vi "Get Arguments.vi"(7 "Function Name":string, 8 "Error In":errorcluster, 11 "OPI Ref":refnum<data-value>) -> (0 "Error Out":errorcluster, 1 "Args Array":string[][](array[string]), 3 "OPI Ref":refnum<data-value>)   [LabVIEW 2012, in "OPI.lvclass"]
doc: "Get the arguments defined for a function. \n\nThe arguments are provided in the format of valid pythonic declaration and 2D array of strings representing argument and pythonic value pairs.\n\n You can keep these representation to reuse them or call them on the PES. This way you can quickly switch between predefined value sets."
uses:
  OPI.lvclass
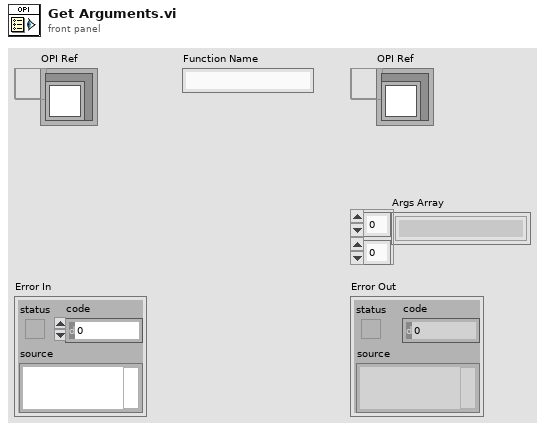
[diagram p1: front panel]
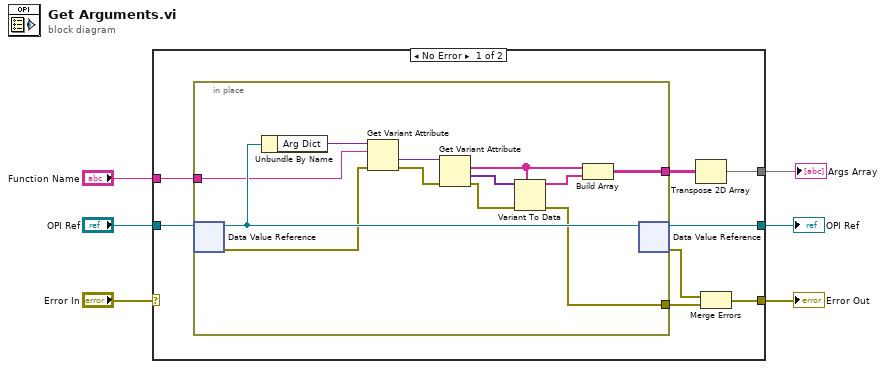
[diagram p0: block diagram]
diagram:
  n1 = case shown="No Error" "Error In" {
    selector: "Error In" -> [_ w27]
    tunnel: "OPI Ref" -> [w14 _]
    tunnel: "Function Name" -> [w13 _]
    tunnel: [w7 _] -> w3
    tunnel: [w9 w27] -> w2
    tunnel: [w8 _] -> w1
    frame No Error {
      n2 = in-place {
        in-place-border: w13 -> [w22]
        in-place-border: [w19] -> w12
        in-place-border: [w17] -> w11
        n3 = in-place-dvr #1(w14) -> (w26:refnum<class "OPI.lvclass">, w18:errorcluster)
        n4 = Unbundle By Name(w26) -> ("Arg Dict"=w23:variant)
        n5 = Get Variant Attribute(Variant=w23, name=w22, error in=w18) -> (value=w24:variant, error out=w25:errorcluster)  [unwired: 1 in, 2 out]
        n6 = Get Variant Attribute(Variant=w24, error in=w25) -> (names=w16:string[], values=w21:variant[], error out=w20:errorcluster)  [unwired: 2 in, 1 out]
        n7 = Variant To Data(error in=w20, type=w16, Variant=w21) -> (data=w15:string[], error out=w17:errorcluster)
        n8 = Build Array(w16, w15) -> (w19:string[][])
        n9 = in-place-dvr #1(w26) -> (w8:refnum<data-value>, w10:errorcluster)
      }
      n10 = Transpose 2D Array(2D array=w12) -> (transposed array=w7:string[][])
      n11 = Merge Errors(w10, w11) -> (w9:errorcluster)
    }
    frame Error {
    }
  }
  "Error Out" <- w2
  "OPI Ref" <- w1
  "Args Array" <- w3
